vi "RFP_Table_Global.vi"() -> ()   [LabVIEW 2018]
panel:
  in  "RFP Table":string[][](array[string])
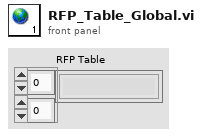
[diagram p1: front panel]
diagram:
